vi "load target hierarchy.vi"(8 "error in":errorcluster, 11 "target hierarchy":T3) -> (0 "error out":errorcluster, 3 "targets cluster out":T1)   [LabVIEW 2013, in "PL_Serialization Interface.lvlib"]
doc: "Takes a flattened instance hierarchy and loads it with the assumption that the root element is of the Target class. If this is incorrect, the process will fail. As part of the load process, this function unflattens the instance data associated with every child of the target, recursively. Since targets have defined structures, the unflattened configurations are then converted into the target/engine/module levels used by the framework."
uses:
  PL_Serialization Interface.lvlib
  <vilib>/NI/Configuration Framework/tree serializer/flat hierarchy.ctl
  <vilib>/NI/Configuration Framework/tree serializer/full hierarchy.ctl
  <vilib>/NI/Configuration Framework/tree serializer/hierarchy element.ctl
  <vilib>/NI/Configuration Framework/tree serializer/instance data.ctl
  platypus configuration/targets cluster.ctl
  target configuration/PL_Target Configuration.lvclass
  platypus configuration/engines cluster.ctl
  <vilib>/NI/Module Execution Interface/Engine Configuration/engine configuration.lvclass
  <vilib>/NI/Tag Bus Module Framework/module configuration/TBM module configuration.lvclass
  <vilib>/NI/Configuration Framework/serializable configuration/NISE_CEF_serializable configuration.lvclass/NISE_CEF_serializable configuration.ctl
  <vilib>/NI/Configuration Framework/serializable configuration/NISE_CEF_serializable configuration.lvclass
  <vilib>/NI/Configuration Framework/tree serializer/NISE_CEF_TreeSerializer.lvlib
  platypus configuration/PLConfigurationSerializer.lvlib
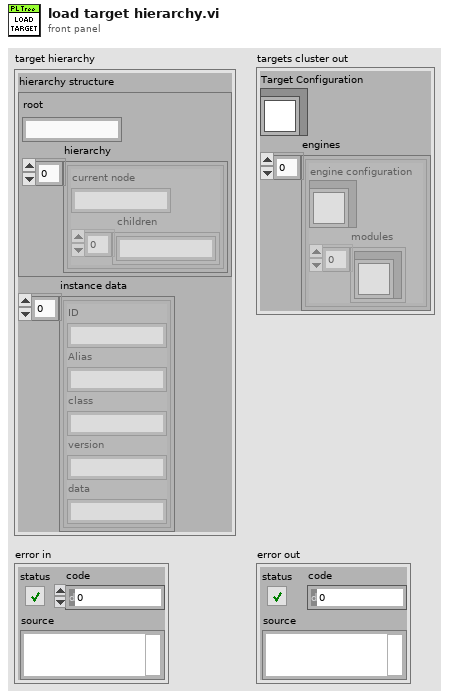
[diagram p1: front panel]
types:
  T1 = typedef "PLConfigurationSerializer.lvlib/targets cluster.ctl" = cluster{"Target Configuration":refnum<class "PL_Target Configuration.lvclass">, "engines":T2[]}
  T2 = typedef "PLConfigurationSerializer.lvlib/engines cluster.ctl" = cluster{"engine configuration":refnum<class "engine configuration.lvclass">, "modules":refnum<class "TBM module configuration.lvclass">[]}
  T3 = typedef "NISE_CEF_TreeSerializer.lvlib/flat hierarchy.ctl" = cluster{"hierarchy structure":T4, "instance data":T6[]}
  T4 = typedef "NISE_CEF_TreeSerializer.lvlib/full hierarchy.ctl" = cluster{"root":string, "hierarchy":T5[]}
  T5 = typedef "NISE_CEF_TreeSerializer.lvlib/hierarchy element.ctl" = cluster{"current node":string, "children":string[]}
  T6 = typedef "NISE_CEF_TreeSerializer.lvlib/instance data.ctl" = cluster{"ID":string, "Alias":string, "class":string, "version":string, "data":string}
  T7 = typedef "NISE_CEF_TreeSerializer.lvlib/memory hierarchy.ctl" = cluster{"hierarchy structure":T4, "instance data":refnum<class "NISE_CEF_serializable configuration.lvclass">[]}
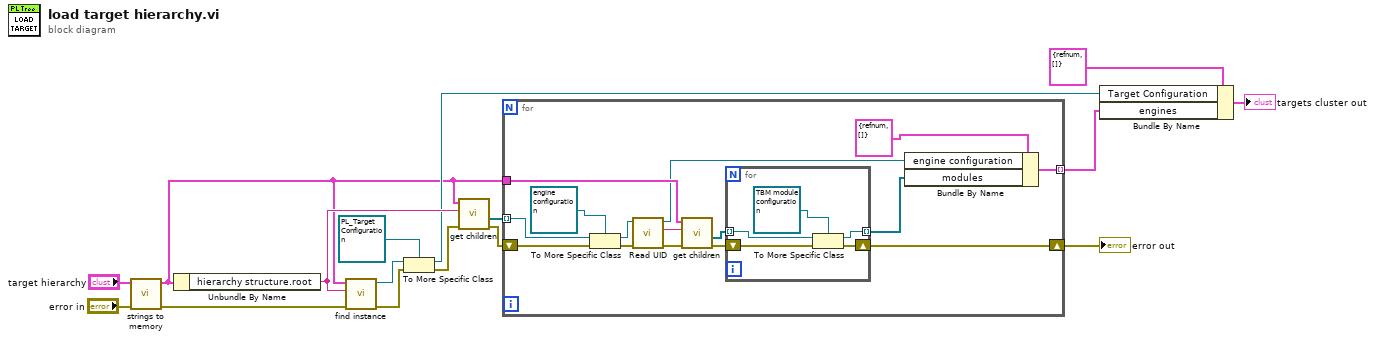
[diagram p0: block diagram]
diagram:
  n1 = call <vilib>:"strings to memory.vi"("error in"="error in", "1.0.0"="target hierarchy") -> ("error out"=w6:errorcluster, "memory hierarchy"=w2:T7)  [unwired: 8 in]
  n2 = Unbundle By Name(w2) -> ("hierarchy structure.root"=w12:string)
  n3 = call <vilib>:"find instance.vi"("error in"=w6, "ID"=w12, "memory hierarchy"=w2) -> ("error out"=w11:errorcluster, "configuration"=w9:refnum<class "NISE_CEF_serializable configuration.lvclass">)  [unwired: 7 in]
  n4 = To More Specific Class(target class=refnum<class "PL_Target Configuration.lvclass"> refnum ("Target Configuration"), reference=w9, error in=w11) -> (specific class reference=w7:refnum<class "PL_Target Configuration.lvclass">, error out=w10:errorcluster)
  n5 = call <vilib>:"get children.vi"("error in"=w10, "ID"=w12, "memory hierarchy"=w2) -> ("error out"=w5:errorcluster, "children"=w4:refnum<class "NISE_CEF_serializable configuration.lvclass">[])  [unwired: 7 in]
  n6 = for {
    tunnel: w4 -> [w31] mode=indexing
    shift-right: [w17] -> w1
    shift-left: w5 -> [w30]
    tunnel: [w27] -> w3 mode=indexing
    tunnel: w2 -> [w23]
    n7 = To More Specific Class(target class=refnum<class "engine configuration.lvclass"> refnum ("engine configuration"), reference=w31, error in=w30) -> (specific class reference=w25:refnum<class "engine configuration.lvclass">, error out=w26:errorcluster)
    n8 = call <vilib>:"Read UID.vi"("error in"=w26, "configuration in"=w25) -> ("error out"=w24:errorcluster, "instance id"=w22:string, "configuration out"=w18:refnum<class "engine configuration.lvclass">)  [unwired: 7 in]
    n9 = call <vilib>:"get children.vi"("error in"=w24, "ID"=w22, "memory hierarchy"=w23) -> ("error out"=w21:errorcluster, "children"=w20:refnum<class "NISE_CEF_serializable configuration.lvclass">[])  [unwired: 7 in]
    n10 = for {
      shift-right: [w32] -> w17
      shift-left: w21 -> [w36]
      tunnel: w20 -> [w35] mode=indexing
      tunnel: [w33] -> w19 mode=indexing
      n11 = To More Specific Class(target class=refnum<class "TBM module configuration.lvclass"> refnum ("module configuration"), reference=w35, error in=w36) -> (specific class reference=w33:refnum<class "TBM module configuration.lvclass">, error out=w32:errorcluster)
    }
    n12 = Bundle By Name(cluster=T2 {"engine configuration"=refnum, "modules"=[]} ("engines cluster"), "engine configuration"=w18, "modules"=w19) -> (w27:T2)
  }
  "error out" <- w1
  n13 = Bundle By Name(cluster=T1 {"Target Configuration"=refnum, "engines"=[]} ("targets cluster out"), "Target Configuration"=w7, "engines"=w3) -> (→"targets cluster out":T1)
